vi "[Template]_ASCII String To Data.vi"(6 "Data Type":T1, 8 "error in (no error)":errorcluster, 11 "Values":string[](array[string])) -> (0 "error out":errorcluster, 2 "Data":i32[][](array[numeric]))   [LabVIEW 2020, in "Current Value Table(Rebuild).lvlib"]
doc: "This VI converts data stored on disk as an ascii string into the correct data type. This VI must perform the opposite operation to the DataToASCIIString function."
uses:
  Current Value Table(Rebuild).lvlib
  Array of I32_Type To Enum.vi
  [Template]_Datatype.ctl
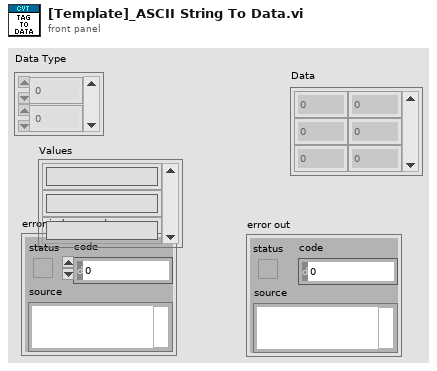
[diagram p1: front panel]
types:
  T1 = typedef "Current Value Table(Rebuild).lvlib/[Template]_Datatype.ctl" = i32[]
  T2 = typedef "Current Value Table(Rebuild).lvlib/Data Types.ctl" = enum16{"Double", "Single", "I64", "I32", "I16", "I8", "U64", "U32", "U16", "U8", "String", "Boolean", "Array of U8", "Array of U16", "Array of U32", "Array of U64", "Array of I64", "Array of I32", "Array of I16", "Array of I8", "Array of Double", "Array of Single", "Array of Boolean", "Array of String"}
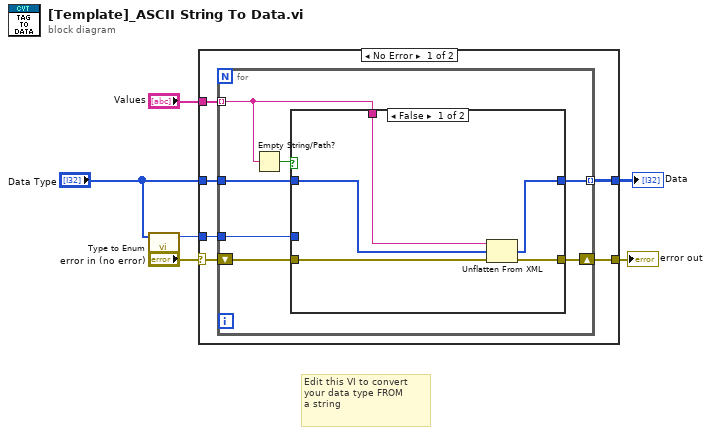
[diagram p0: block diagram]
diagram:
  # "Edit this VI to convert\nyour data type FROM\na string"
  n1 = call-poly "Type to Enum.vi"("Default"="Data Type") -> ("Data Type Enum"=w2:T2)  [unwired: 10 in]
  n2 = case shown="No Error" "error in (no error)" {
    selector: "error in (no error)" -> [w10 w27]
    tunnel: "Data Type" -> [w12 _]
    tunnel: "Values" -> [w11 _]
    tunnel: [w9 w27] -> w4
    tunnel: [w8 _] -> w3
    tunnel: w2 -> [w7 _]
    frame No Error {
      n3 = for {
        tunnel: w12 -> [w19]
        tunnel: w11 -> [w18] mode=indexing
        shift-right: [w13] -> w9
        shift-left: w10 -> [w15]
        tunnel: [w16] -> w8 mode=indexing
        tunnel: w7 -> [w14]
        n4 = Empty String/Path?(string/path=w18) -> (empty?=w17:bool)
        n5 = case shown="False" w17 {
          tunnel: w19 -> [w22 w26]
          tunnel: w18 -> [w21 _]
          tunnel: [w20 w26] -> w16
          tunnel: w15 -> [w23 w25]
          tunnel: w14 -> [_ _]
          tunnel: [w24 w25] -> w13
          frame False {
            n6 = Unflatten From XML(xml string=w21, type=w22, error in (no error)=w23) -> (value=w20:T1, error out=w24:errorcluster)
          }
          frame True {
          }
        }
      }
    }
    frame Error {
    }
  }
  "error out" <- w4
  "Data" <- w3
